vi "Calculate Saccade Parameters.vi"(7 "Impulse Data":refnum<data-value>, 8 "error in (no error)":errorcluster, 9 "Sample Rate (Hz)":dbl, 10 "enum_direction":enum16{"Positive", "Negative"}(ring) caption="Impulse Direction", 11 "Saccades in":T1[](array[typedef])) -> (0 "error out":errorcluster, 3 "Saccade out":T1[](array[typedef]))   [LabVIEW 2016]
uses:
  Type Definitions/Saccade Analyser Saccade Data.ctl
  Type Definitions/Saccade Analyser Impulse Data.ctl
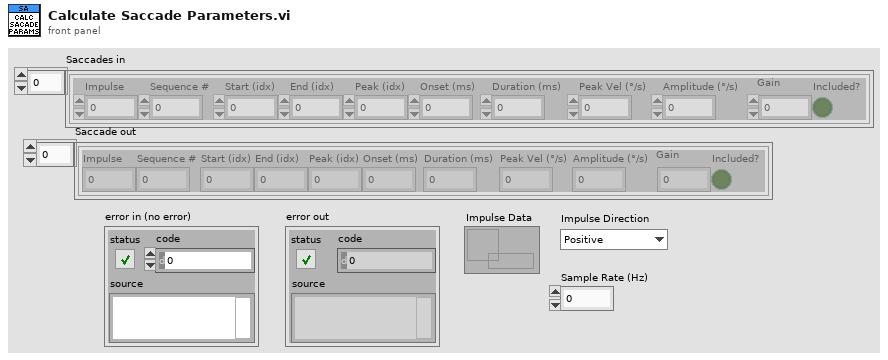
[diagram p1: front panel]
types:
  T1 = typedef "Saccade Analyser Saccade Data.ctl" = cluster{"Impulse":i32, "Sequence #":dbl, "Start (idx)":dbl, "End (idx)":dbl, "Peak (idx)":dbl, "Onset (ms)":dbl, "Duration (ms)":dbl, "Peak Vel (°/s)":dbl, "Amplitude (°/s)":dbl, "Gain":dbl, "Included?":bool}
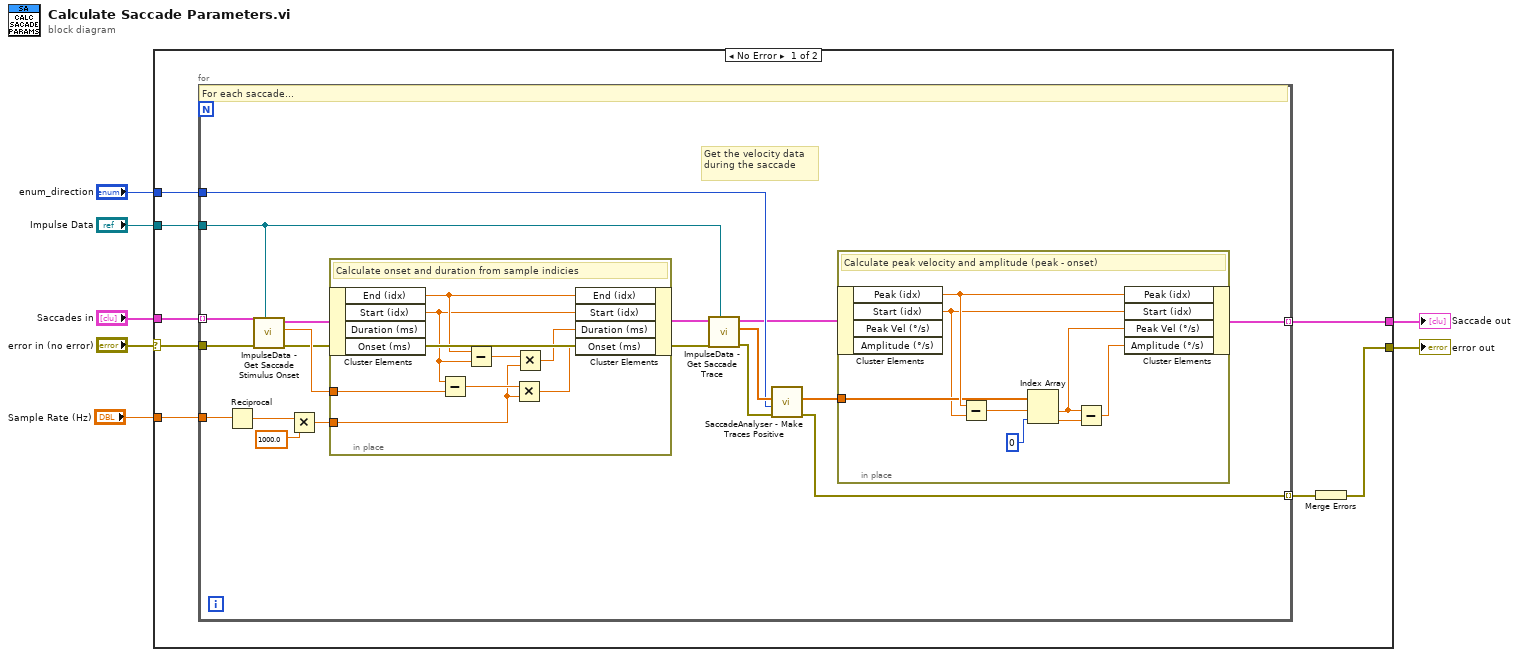
[diagram p0: block diagram]
diagram:
  n1 = case shown="No Error" "error in (no error)" {
    selector: "error in (no error)" -> [w13 w50]
    tunnel: "Saccades in" -> [w15 w51]
    tunnel: [w8 w51] -> w4
    tunnel: [w10 w50] -> w6
    tunnel: "Impulse Data" -> [w14 _]
    tunnel: "enum_direction" -> [w12 _]
    tunnel: "Sample Rate (Hz)" -> [w9 _]
    frame No Error {
      n2 = for {
        tunnel: w15 -> [w31] mode=indexing
        tunnel: w14 -> [w19]
        tunnel: w13 -> [w30]
        tunnel: w12 -> [w22]
        tunnel: [w18] -> w11 mode=indexing
        tunnel: w9 -> [w17]
        tunnel: [w16] -> w8 mode=indexing
        # "Get the velocity data during the saccade"
        # "For each saccade..."
        n3 = Reciprocal(x=w17) -> (1/x=w33:dbl)
        n4 = call "ImpulseData - Get Saccade Stimulus Onset.vi"("Saccade in"=w31, "error in (no error)"=w30, "Impulse Data"=w19) -> ("Saccade out"=w29:T1, "Onset (idx)"=w28:dbl, "error out"=w23:errorcluster)  [unwired: 4 in, 1 out]
        n5 = Multiply(x=w33, y=1000.0) -> (x*y=w27:dbl)
        n6 = in-place {
          in-place-border: w28 -> [w45]
          in-place-border: w27 -> [w42]
          # "Calculate onset and duration from sample indicies"
          n7 = in-place-cluster #1(w29) -> ("End (idx)"=w47:dbl, "Start (idx)"=w46:dbl)  [unwired: 2 out]
          n8 = Subtract(x=w46, y=w45) -> (x-y=w48:dbl)
          n9 = Subtract(x=w47, y=w46) -> (x-y=w49:dbl)
          n10 = Multiply(x=w48, y=w42) -> (x*y=w43:dbl)
          n11 = Multiply(x=w49, y=w42) -> (x*y=w44:dbl)
          n12 = in-place-cluster #1("End (idx)"=w47, "Start (idx)"=w46, "Duration (ms)"=w44, "Onset (ms)"=w43) -> (w24:T1)
        }
        n13 = call "ImpulseData - Get Saccade Trace.vi"("Saccade in"=w24, "error in (no error)"=w23, "Impulse Data"=w19) -> ("Saccade out"=w21:T1, "Response Data"=w25:dbl[], "error out"=w26:errorcluster)  [unwired: 4 in, 1 out]
        n14 = call "SaccadeAnalyser - Make Traces Positive.vi"("error in (no error)"=w26, "enum_direction"=w22, "Response in"=w25) -> ("error out"=w18:errorcluster, "Response out"=w20:dbl[])  [unwired: 6 in, 1 out]
        n15 = in-place {
          in-place-border: w20 -> [w35]
          # "Calculate peak velocity and amplitude (peak - onset)"
          n16 = in-place-cluster #2(w21) -> ("Peak (idx)"=w38:dbl, "Start (idx)"=w34:dbl)  [unwired: 2 out]
          n17 = Subtract(x=w38, y=w34) -> (x-y=w37:dbl)
          n18 = Index Array(array=w35, index #1=w37, index #2=0 ("index")) -> (element #1=w41:dbl, element #2=w40:dbl)
          n19 = Subtract(x=w41, y=w40) -> (x-y=w39:dbl)
          n20 = in-place-cluster #2("Peak (idx)"=w38, "Start (idx)"=w34, "Peak Vel (°/s)"=w41, "Amplitude (°/s)"=w39) -> (w16:T1)
        }
      }
      n21 = Merge Errors(w11) -> (w10:errorcluster)
    }
    frame Error {
    }
  }
  "error out" <- w6
  "Saccade out" <- w4
